vi "create.vi"(8 "error in (no error)":errorcluster, 11 "MulticolumnListbox in":refnum<vi>) -> (0 "error out":errorcluster, 3 "TransactionListUserInterface out":refnum<class "TransactionListUserInterface.lvclass">)   [LabVIEW 2018, in "TransactionListUserInterface.lvclass"]
uses:
  TransactionListUserInterface.lvclass
  TransactionListUserInterface.lvclass/TransactionListUserInterface.ctl
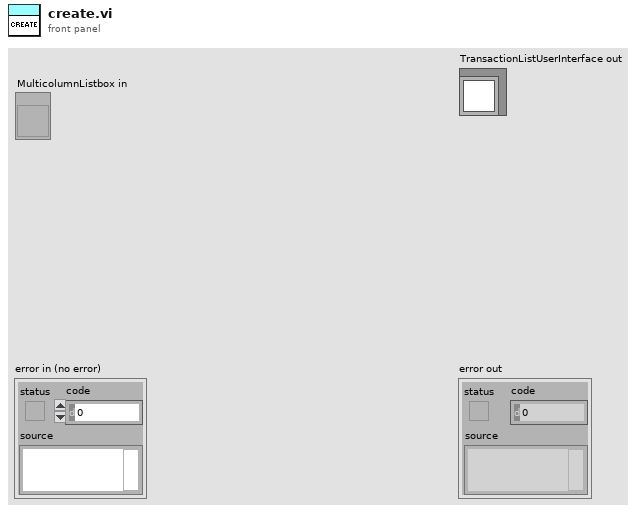
[diagram p1: front panel]
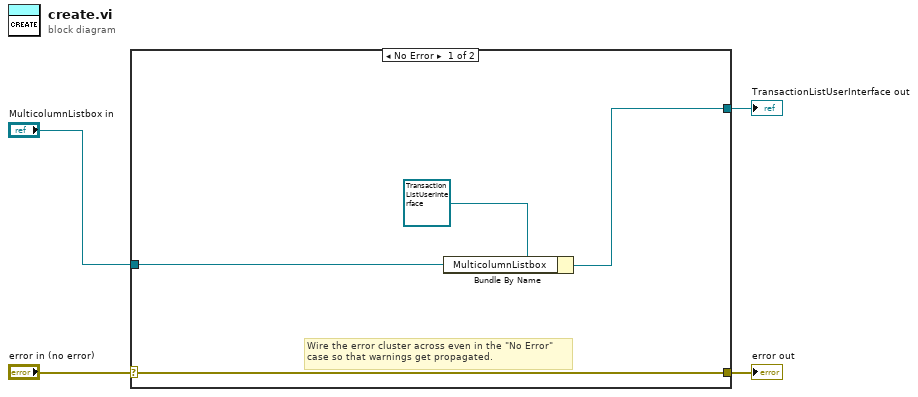
[diagram p0: block diagram]
diagram:
  n1 = case shown="No Error" "error in (no error)" {
    selector: "error in (no error)" -> [w8 w9]
    tunnel: [w8 w9] -> w3
    tunnel: [w6 _] -> w2
    tunnel: "MulticolumnListbox in" -> [w5 _]
    frame No Error {
      # "Wire the error cluster across even in the \"No Error\"\ncase so that warnings get propagated."
      n2 = Bundle By Name(cluster=refnum<class "TransactionListUserInterface.lvclass"> refnum ("TransactionListUserInterface.lvclass"), "MulticolumnListbox"=w5) -> (w6:refnum<class "TransactionListUserInterface.lvclass">)
    }
    frame Error {
    }
  }
  "error out" <- w3
  "TransactionListUserInterface out" <- w2
